vi "AudioStreamer.ProcessVoice.vi"(0 "State in":T1, 7 "Queue in":refnum<queue>, 9 "ptsPerFrame":i32) -> (4 "State out":T1, 8 "Array":dbl[](array[numeric]))   [LabVIEW 2020]
uses:
  Test VIs/AudioStreamer.VoiceState.ctl
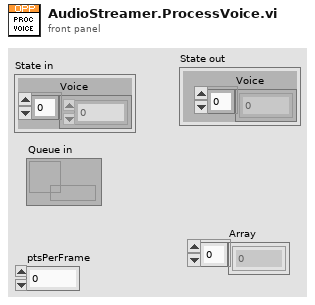
[diagram p1: front panel]
types:
  T1 = typedef "AudioStreamer.VoiceState.ctl" = cluster{"Voice":dbl[]}
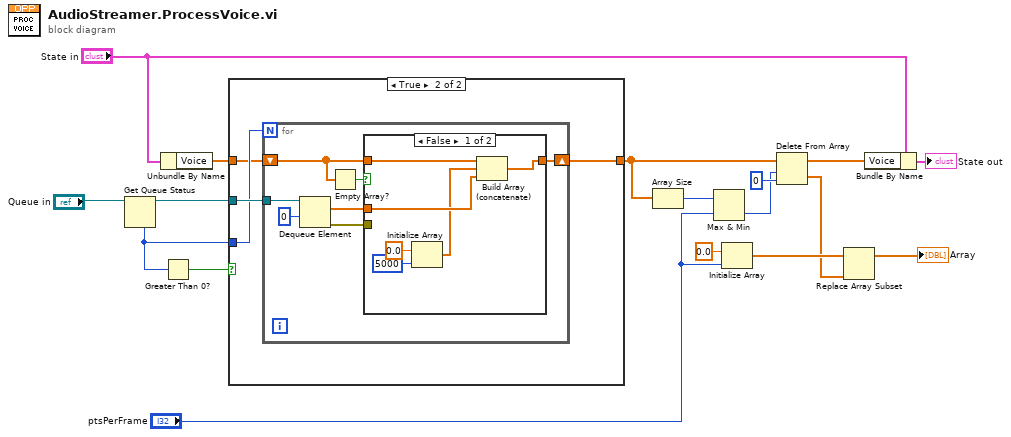
[diagram p0: block diagram]
diagram:
  n1 = Get Queue Status(queue="Queue in") -> (queue out=w14:refnum<queue>, # elements in queue=w13:i32)  [unwired: 2 in, 6 out]
  n2 = Unbundle By Name("State in") -> ("Voice"=w15:dbl[])
  n3 = Greater Than 0?(x=w13) -> (x > 0?=w16:bool)
  n4 = case shown="True" w16 {
    tunnel: w15 -> [w18 w20]
    tunnel: w14 -> [_ w22]
    tunnel: w13 -> [_ w21]
    tunnel: [w18 w19] -> w7
    frame False {
    }
    frame True {
      n5 = for {
        N: w21 -> [_]
        tunnel: w22 -> [w29]
        shift-right: [w23] -> w19
        shift-left: w20 -> [w25]
        n6 = Dequeue Element(queue=w29, timeout in ms (-1)=0) -> (element=w26:dbl[], error out=w27:errorcluster)  [unwired: 1 in, 2 out]
        n7 = Empty Array?(array=w25) -> (empty?=w24:bool)
        n8 = case shown="False" w24 {
          tunnel: w25 -> [w35 _]
          tunnel: w27 -> [_ _]
          tunnel: w26 -> [w31 w36]
          tunnel: [w34 w36] -> w23
          frame False {
            n9 = Initialize Array(0.0 ("element"), 5000 ("dimension size")) -> (w30:dbl[])
            n10 = Build Array (concatenate)(w35, w30, w31) -> (w34:dbl[])
          }
          frame True {
          }
        }
      }
    }
  }
  n11 = Array Size(array=w7) -> (size(s)=w9:i32)
  n12 = Max & Min(x=w9, y="ptsPerFrame") -> (min(x,y)=w5:i32)  [unwired: 1 out]
  n13 = Initialize Array(0.0 ("element"), "ptsPerFrame") -> (w11:dbl[])
  n14 = Delete From Array(array=w7, length=w5, index=0) -> (deleted portion=w4:dbl[], array with subset deleted=w2:dbl[])
  n15 = Replace Array Subset(array=w11, new element=w4) -> (→"Array":dbl[])  [unwired: 1 in]
  n16 = Bundle By Name(cluster="State in", "Voice"=w2) -> (→"State out":T1)
